vi "User Event Init.vi"(0 "init?":bool) -> (6 "main menu User Event":refnum<user-event>, 10 "Event Registration Refnum":refnum<event-registration>)   [LabVIEW 2021]
uses:
  Sub Controls/User Event Message.ctl
  Sub Controls/User Event Command.ctl
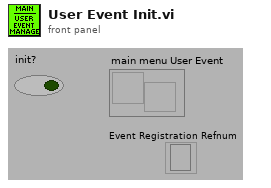
[diagram p1: front panel]
types:
  T1 = typedef "User Event Message.ctl" = cluster{"Command":T2}
  T2 = typedef "User Event Command.ctl" = enum32{"Stop Config"}
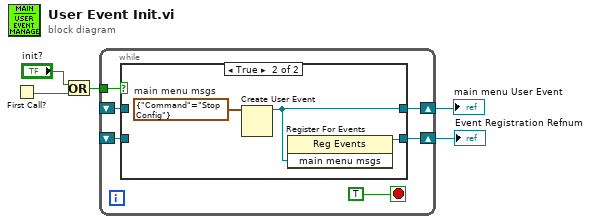
[diagram p0: block diagram]
diagram:
  n1 = First Call?() -> (First Call?: T/F=w5:bool)
  n2 = Or(x="init?", y=w5) -> (x .or. y?=w3:bool)
  n3 = while {
    shift-right: [w11] -> w1
    shift-left: _ -> [w9]
    tunnel: w3 -> [w10]
    shift-right: [w7] -> w2
    shift-left: _ -> [w6]
    stop <- TRUE stop-if-true
    n4 = case shown="True" w10 {
      tunnel: [w13 w15] -> w11
      tunnel: w9 -> [w13 _]
      tunnel: [w12 w14] -> w7
      tunnel: w6 -> [w12 _]
      frame False {
      }
      frame True {
        w16 = T1 {"Command"=enum."Stop Config"}  # main menu msgs
        n5 = Create User Event(user event datatype=w16) -> (user event=w14:refnum<user-event>)  [unwired: 1 in, 1 out]
        n6 = register-events(w14) -> (reference out=w15:refnum<event-registration>)  [unwired: 2 in, 1 out]
      }
    }
  }
  "main menu User Event" <- w2
  "Event Registration Refnum" <- w1
